vi "Set Type.vi"(10 "Type":refnum<class "Type.lvclass">, 11 "StringPanel in":refnum<class "StringPanel.lvclass">) -> (3 "StringPanel out":refnum<class "StringPanel.lvclass">)   [LabVIEW 2020, in "Conditum-Tools.lvlib" / "StringPanel.lvclass"]
uses:
  StringPanel.lvclass
  Conditum-Clone/Columns/Type/Type.lvclass
  StringPanel.lvclass/StringPanel.ctl
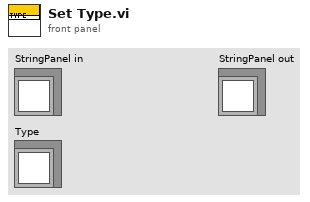
[diagram p1: front panel]
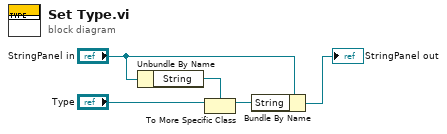
[diagram p0: block diagram]
diagram:
  n1 = Unbundle By Name("StringPanel in") -> ("String"=w4:refnum<class "String.lvclass">)
  n2 = To More Specific Class(target class=w4, reference="Type") -> (specific class reference=w5:refnum<class "String.lvclass">)  [unwired: 1 in, 1 out]
  n3 = Bundle By Name(cluster="StringPanel in", "String"=w5) -> (→"StringPanel out":refnum<class "StringPanel.lvclass">)
